vi "Exercise 3-6.vi"() -> ()   [LabVIEW 2014]
panel:
  in  "stop":bool
  out "New Temperature":dbl
  in  "Conversion":T1(ring)
  in  "Temperature":dbl
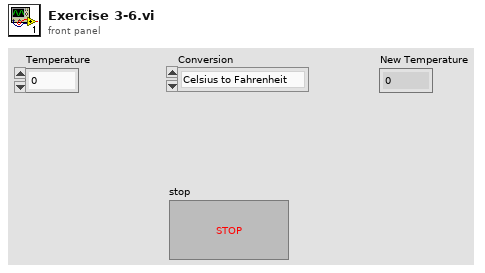
[diagram p1: front panel]
types:
  T1 = enum16{"Celsius to Fahrenheit", "Fahrenheit to Celsius", "Celsius to Kelvin", "Fahrenheit to Kelvin"}
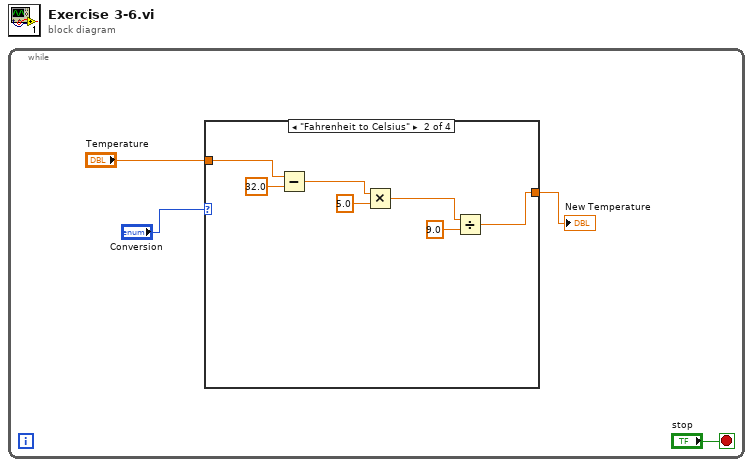
[diagram p0: block diagram]
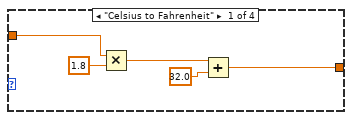
[diagram p2: hidden frame]
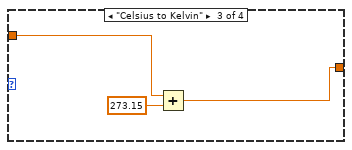
[diagram p3: hidden frame]
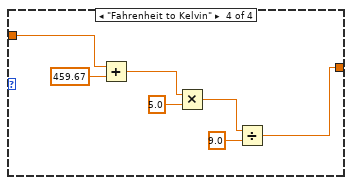
[diagram p4: hidden frame]
diagram:
  n1 = while {
    stop <- "stop" stop-if-true
    n2 = case shown="\"Fahrenheit to Celsius\"" "Conversion" {
      tunnel: [w7 w11 w17 w20] -> w3
      tunnel: "Temperature" -> [w5 w10 w18 w25]
      frame "Celsius to Fahrenheit" {
        n3 = Multiply(x=w5, y=1.8) -> (x*y=w6:dbl)
        n4 = Add(x=w6, y=32.0) -> (x+y=w7:dbl)
      }
      frame "Fahrenheit to Celsius" {
        n5 = Subtract(x=w10, y=32.0) -> (x-y=w14:dbl)
        n6 = Multiply(x=w14, y=5.0) -> (x*y=w12:dbl)
        n7 = Divide(x=w12, y=9.0) -> (x/y=w11:dbl)
      }
      frame "Celsius to Kelvin" {
        n8 = Add(x=w18, y=273.15) -> (x+y=w17:dbl)
      }
      frame "Fahrenheit to Kelvin" {
        n9 = Add(x=w25, y=459.67) -> (x+y=w24:dbl)
        n10 = Multiply(x=w24, y=5.0) -> (x*y=w23:dbl)
        n11 = Divide(x=w23, y=9.0) -> (x/y=w20:dbl)
      }
    }
    "New Temperature" <- w3
  }
